vi "Arduino Writer.vi"(11 "Start Of Match":bool) -> ()   [LabVIEW 2014]
panel:
  # "Remember: STOP before unplugging\nARDUINO!!!!!"
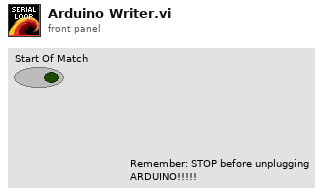
[diagram p1: front panel]
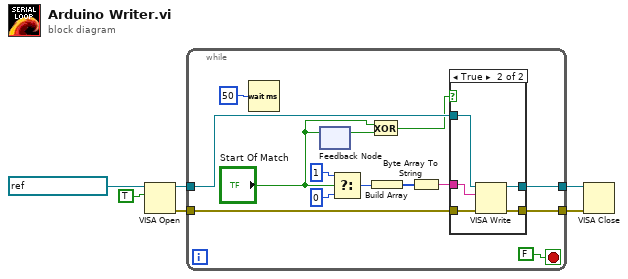
[diagram p0: block diagram]
diagram:
  n1 = VISA Open(duplicate session (F)=TRUE, VISA resource name=refnum<visa-resource-name> "ASRL3::INSTR") -> (VISA resource name=w3:refnum<visa-resource-name>, error out=w2:errorcluster)  [unwired: 1 in, 2 out]
  n2 = while {
    tunnel: w3 -> [w20]
    tunnel: [w18] -> w6
    tunnel: w2 -> [w16]
    tunnel: [w15] -> w5
    stop <- FALSE stop-if-true
    n3 = Wait (ms)(milliseconds to wait=u32 50) -> ()  [unwired: 1 out]
    n4 = feedback #1() -> (w8:bool)  [unwired: 1 in]
    n5 = feedback-in #1("Start Of Match") -> ()
    n6 = Select(t=u8 1 ("element"), s="Start Of Match", f=u8 0) -> (s? t:f=w14:u8)
    n7 = Exclusive Or(1:w8, 2:"Start Of Match") -> (0:w9:bool)
    n8 = Build Array(w14) -> (w11:u8[])
    n9 = Byte Array To String(unsigned byte array=w11) -> (string=w19:string)
    n10 = case shown="True" w9 {
      tunnel: w20 -> [w22 w27]
      tunnel: w19 -> [_ w26]
      tunnel: [w22 w25] -> w18
      tunnel: w16 -> [w21 w24]
      tunnel: [w21 w23] -> w15
      frame False {
      }
      frame True {
        n11 = VISA Write(VISA resource name=w27, write buffer=w26, error in (no error)=w24) -> (VISA resource name out=w25:refnum<visa-resource-name>, error out=w23:errorcluster)  [unwired: 1 out]
      }
    }
  }
  n12 = VISA Close(VISA resource name=w6, error in (no error)=w5) -> ()  [unwired: 1 out]
